vi "PseudoInverse Matrix.vi"   [LabVIEW 2024, in "NI_AALPro.lvlib"]
doc: "<p>Finds the <strong>PseudoInverse Matrix</strong> of <strong>Input Matrix</strong>. Wire data to the <strong>Input Matrix</strong> input to determine the polymorphic instance to use or <a href=\"nihelplauncher://docs/csh?context=lvcore_lvhowto_selectingdefaultinstpolyvi\">manually select</a> the instance.\n</p>"
uses:
  NI_AALPro.lvlib
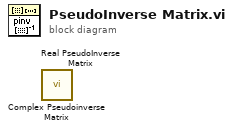
[diagram p0: block diagram]
diagram:
  n1 = call "Complex Pseudoinverse Matrix.vi"() -> ()  [unwired: 2 in, 2 out]
  n2 = call "Real PseudoInverse Matrix.vi"() -> ()  [unwired: 2 in, 2 out]
